vi "Read TIFF.vi"(8 "error in (no error)":errorcluster, 10 "Path":path, 11 "ImageHandler in":refnum<class "ImageHandler.lvclass">) -> (0 "error out":errorcluster, 3 "ImageHandler out":refnum<class "ImageHandler.lvclass">)   [LabVIEW 2021, in "ImageHandler.lvlib" / "ImageHandler.lvclass"]
uses:
  ImageHandler.lvclass
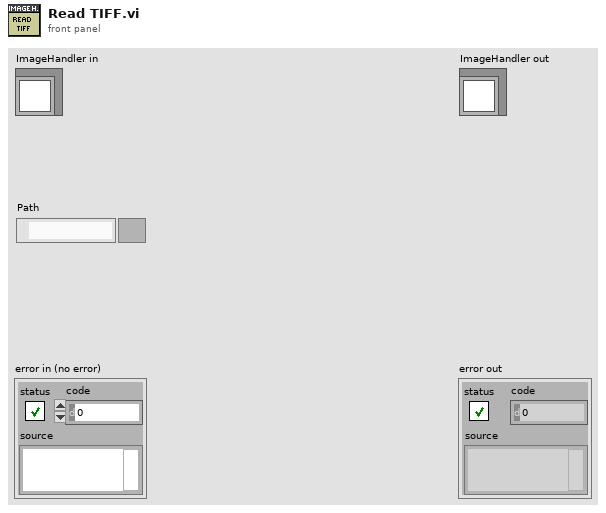
[diagram p1: front panel]
types:
  T1 = typedef "IMAQ Image.ctl" = refnum<image>
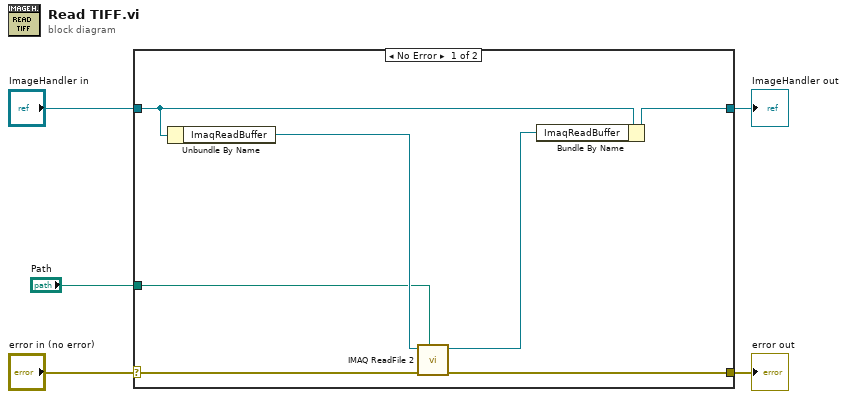
[diagram p0: block diagram]
diagram:
  n1 = case shown="No Error" "error in (no error)" {
    selector: "error in (no error)" -> [w12 w14]
    tunnel: [w11 w14] -> w4
    tunnel: [w7 w13] -> w2
    tunnel: "ImageHandler in" -> [w8 w13]
    tunnel: "Path" -> [w9 _]
    frame No Error {
      n2 = Unbundle By Name(w8) -> ("ImaqReadBuffer"=w10:T1)
      n3 = call "IMAQ ReadFile 2"("File Path"=w9, "error in (no error)"=w12, "Image"=w10) -> ("error out"=w11:errorcluster, "Image Out"=w6:T1)  [unwired: 4 in, 3 out]
      n4 = Bundle By Name(cluster=w8, "ImaqReadBuffer"=w6) -> (w7:refnum<class "ImageHandler.lvclass">)
    }
    frame Error {
    }
  }
  "error out" <- w4
  "ImageHandler out" <- w2
